vi "SendPluginActivatedEvent.vi"(8 "error in (no error)":errorcluster, 11 "_LVCMPlugin in":refnum<class "GCMPlugin.lvclass">) -> (0 "error out":errorcluster, 3 "_LVCMPlugin out":refnum<class "GCMPlugin.lvclass">)   [LabVIEW 2014, in "GCMPlugin.lvclass"]
uses:
  GCMPlugin/GCMPlugin.lvclass
  <vilib>/event_ctls.llb/usereventprio.ctl
  GCMPlugin/GCMPlugin.lvclass/GCMPlugin.ctl
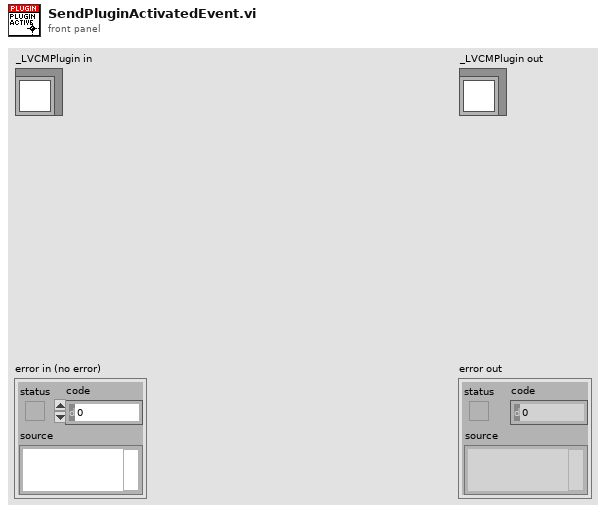
[diagram p1: front panel]
types:
  T1 = typedef "usereventprio.ctl" = enum32{"high priority", "normal priority"}
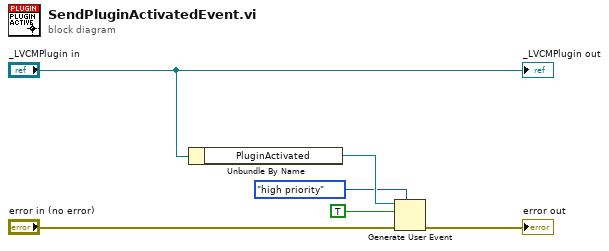
[diagram p0: block diagram]
diagram:
  n1 = Unbundle By Name("_LVCMPlugin in") -> ("PluginActivated"=w3:refnum<user-event>)
  n2 = Generate User Event(priority (normal)=usereventprio."high priority", user event=w3, event data cluster=TRUE ("event data"), error in="error in (no error)") -> (error out=→"error out":errorcluster)  [unwired: 1 out]
  "_LVCMPlugin out" <- "_LVCMPlugin in"
